vi "Protocol.J1939 Filter by Device Address.vi"(8 "error in":errorcluster, 9 "Active Request?":bool, 10 "CAN Frame":T5 {"payload" format="%x"; "timestamp" format="%<%.7X\n%x>T"; "type" items=["CAN Data"=0, "CAN Remote"=1, "CAN Bus Error"=2, "CAN 2.0 Data"=8, "CAN FD Data"=16, "CAN FD+BRS Data"=24, "J1939 Data"=192, "Delay"=224, "Log Trigger"=225, "Start Trigger"=226]; "identifier" format="%x"}, 11 "J1939 Cluster":T2) -> (0 "error out":errorcluster, 1 "Pass Through":bool, 3 "State":T1=enum."ACL")   [LabVIEW 2019, in "J1939 Addon Engine.lvlib"]
uses:
  J1939 Addon Engine.lvlib
  <vilib>/xnet/xnet.llb/XNET Frame CAN.ctl
  <vilib>/xnet/xnet.llb/XNET Frame Type CAN.ctl
  Types/Protocol.Refs.ctl
  Shared/J1939 Utilities/Types/CAN Outgoing Message Cluster.ctl
  Types/Protocol.RQST Lookup Table Reference.ctl
  Types/Protocol.Address Table Reference.ctl
  Shared/J1939 Utilities/Types/Message Types.ctl
  Shared/J1939 Utilities/J1939 Utilities.lvlib
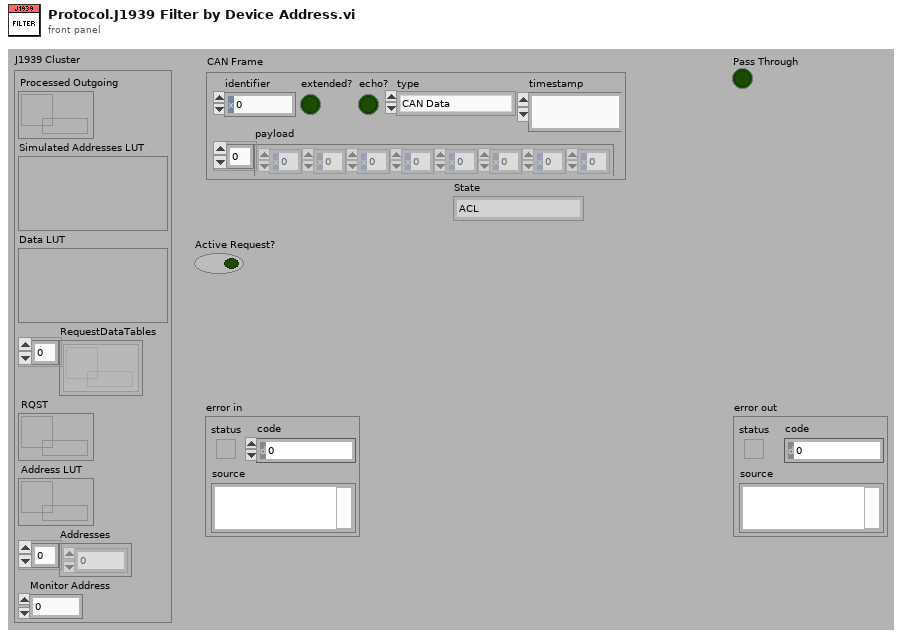
[diagram p1: front panel]
types:
  T1 = typedef "J1939 Addon Shared.lvlib/J1939 Utilities.lvlib/Message Types.ctl" = enum8{"PDU 1", "RQST2", "XFER", "ACKM", "RQST", "TP.DT - RTS/CTS", "TP.DT - BAM", "TP.CM - RTS", "TP.CM - CTS", "TP.CM - EndofMsgACK", "TP.CM - BAM", "TP.CM - Abort", "TP.CM - Error", "ACL", "Proprietary A", "PDU 2", "Proprietary B", "Error"}
  T2 = typedef "J1939 Addon Engine.lvlib/Protocol.Refs.ctl" = cluster{"Processed Outgoing":refnum<queue>, "Simulated Addresses LUT":variant, "Data LUT":variant, "RequestDataTables":refnum<k33>[], "RQST":T3, "Address LUT":T4, "Addresses":u8[], "Monitor Address":u8}
  T3 = typedef "J1939 Addon Engine.lvlib/Protocol.RQST Lookup Table Reference.ctl" = refnum<data-value>
  T4 = typedef "J1939 Addon Engine.lvlib/Protocol.Address Table Reference.ctl" = refnum<data-value>
  T5 = typedef "XNET Frame CAN.ctl" = cluster{"timestamp":timestamp, "payload":u8[], "identifier":u32, "type":T6, "extended?":bool, "echo?":bool}
  T6 = typedef "XNET Frame Type CAN.ctl" = u8
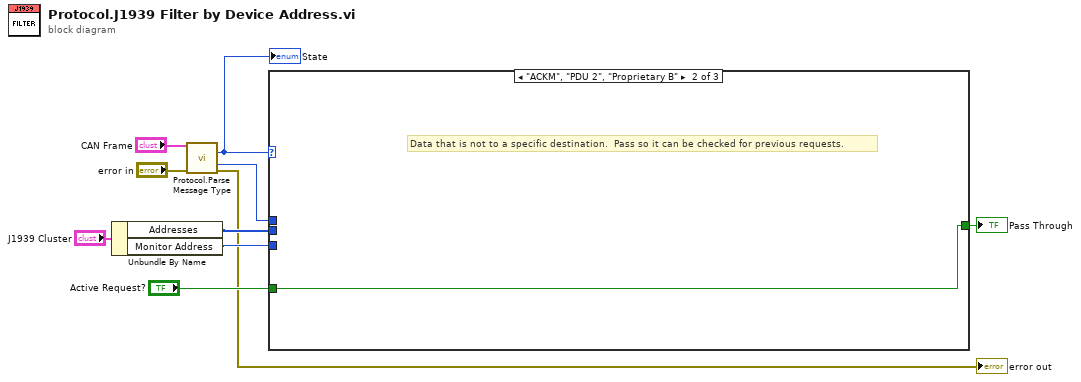
[diagram p0: block diagram]
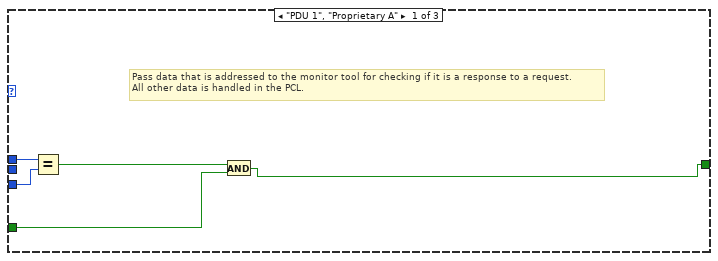
[diagram p2: hidden frame]
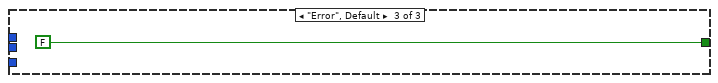
[diagram p3: hidden frame]
diagram:
  n1 = Unbundle By Name("J1939 Cluster") -> ("Addresses"=w4:u8[], "Monitor Address"=w3:u8)
  n2 = call "Protocol.Parse Message Type.vi"("CAN frame"="CAN Frame", "error in"="error in") -> ("State"=w10:T1, "PDU S"=w9:u8, "error out"=→"error out":errorcluster)  [unwired: 11 out]
  "State" <- w10
  n3 = case shown="\"ACKM\", \"PDU 2\", \"Proprietary B\"" w10 {
    tunnel: w4 -> [_ _ _]
    tunnel: w9 -> [w15 _ _]
    tunnel: [w11 w16 FALSE] -> w8
    tunnel: w3 -> [w14 _ _]
    tunnel: "Active Request?" -> [w12 w16 _]
    frame "PDU 1", "Proprietary A" {
      # "Pass data that is addressed to the monitor tool for checking if it is a response to a request.\nAll other data is handled in the PCL."
      n4 = Equal?(x=w15, y=w14) -> (x = y?=w13:bool)
      n5 = And(x=w13, y=w12) -> (x .and. y?=w11:bool)
    }
    frame "ACKM", "PDU 2", "Proprietary B" {
      # "Data that is not to a specific destination.  Pass so it can be checked for previous requests."
    }
    frame "Error", Default {
    }
  }
  "Pass Through" <- w8
